vi "VG_progressBar.vi"() -> ()   [LabVIEW 2020]
panel:
  out "progression":dbl(slide) scale=0.0..1000.0 scale format="%#_6f"
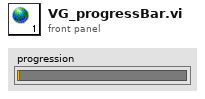
[diagram p1: front panel]
diagram:
